vi "CPP-BLplotter.vi"(0 "Plot Array":cluster{dbl[], dbl[]}[](array[cluster])=[{[500.0, 500.0, 953.54, 215.0, 270.0, 320.0, 445.0, 525.0, 600.0, 675.0, 750.0, 825.0, 900.0, 960.0, 1010.0, 1060.0], [4.614524, 4.54365, 5.818368, 0.1374656, 0.6662545, 1.465458, 3.619824, 4.848976, 5.887329, 5.940571, 6.152151, 5.717487, 5.600293, 5.40069, 5.154843, 5.121789]}, {[100.0, 150.0, 215.0, 270.0, 320.0, 445.0, 525.0, 600.0, 675.0, 750.0, 825.0, 900.0, 960.0, 1010.0, 1060.0], [0.002314715, -0.00693192, 0.120417, 0.6880509, 1.519176, 3.513709, 5.065183, 6.116033, 6.096773, 5.938465, 5.593788, 5.5597, 5.387002, 5.304077, 4.887903]}] {"?" format="%.2f"; "?" format="%.2f"}, 1 "Job Directory":path=path "/G4_2_HD/Users/paulhayden/Documents/Projects/Westlakes_resolution") -> (2 "Saved Automatically?":bool, 3 "gnuplotScript":string="set term epslatex\nset output \"Plot.eps\"\nset xlabel '$Distance~(m)$'\nset ylabel '$DF~(s/m^3)\\times10^6$'\nset samples 1000\nset pointsize 1.00\nset title '$B38~Centreline~Glc$' 0, 0\nset size 0.75,0.9\n\n#set key 450, -2.5833\n unset key\nset label 1 '~~~~~~~~~~~Angle~(deg)~=~0' at -100, -2.58\nset label 2 '~~~~~~~~~~~Height~(m)~=~5' at -100, -3.27\n set xrange [0 : 500] \n# set autoscale x \n set yrange [0.10000 : 7]\n# set autoscale y \n\nplot \"B38_Centreline_Glc.dat\" index 0 using 1:2 axes x1y1 title '$File=B38R~DDD.xls$' with points 1 1, \\\n\"B38_Centreline_Glc.dat\" index 1 using 1:2 axes x1y1 title '$File=B38R~DDD~1.xls$' with points 1 3", 4 "Plot data file":path)   [LabVIEW 2012]
uses:
  Results_plotter_Global.vi
panel:
  in  "Tab Control":enum32{"Good Shit", "Boring Shit"}(tab)
  in  "Cancel Button":bool
  in  "Print Button":bool
  out "Velocity":cluster{dbl[], dbl[]}(graph)
  out "Turbulence":cluster{dbl[], dbl[]}(graph)
  in  "Plot Title":u16(ring) items=["Title String Only", "Number of Measurements", "Measuring:Instrument:Type", "Comments::", "Profile::", "URef::", "ULoc::", "HF:X:(mm)", "HF:Y:(mm)", "HF:Z:(mm)", "HF:DipAngle:Deg", "Uhf/Uref::", "TI:HF:%", "Uhf::", "Var(hf)::", "5HP:X:(mm)", "5HP:Y:(mm)", "5HP:Z:(mm)", "U5hp/Uref::", "V5hp/Uref::", "W5hp/Uref::", "Vmag5hp/Uref::", "TI:U5HP:%", "TI:V5HP:%", "TI:W5HP:%", "TI:Vmag5HP:%", "U_Mean::", "U_SD::", "V_Mean::", "V_SD::", "W_Mean::", "W_SD::", "Vmag_Mean::", "Vmag_SD::", "GoodFraction::", "5HP:P1:mmH2O", "Skew(hf)::", "Kurt(hf)::", "HF:Standard Error:in Mean", "HF:Standard Error:in Variance", "HF:Timescale Estimate:Integrated to 25%", "Reference:Temperature:Used for Corrections", "Atmos:Pressure:Used for Corrections", "Date::", "Multi Run:Start Time:", "Time:Measurement:Commenced", "Seconds:since:1st Jan", "Messages::", "Raw:Data:Filename"]
  in  "Filename Max length":i32=255
  out "Final Title":string="B38 Centreline Glc"
  out "Path":path
  in  "Plot Title Post Block":string
  in  "Plot Title Pre Block":string
  in  "Show Script Editor?":bool
  # "put a load of nice controls here for ref height etc, then a button to say \"print it\" that makes and runs a gnuplot script for \nthe graphs as you have them....."
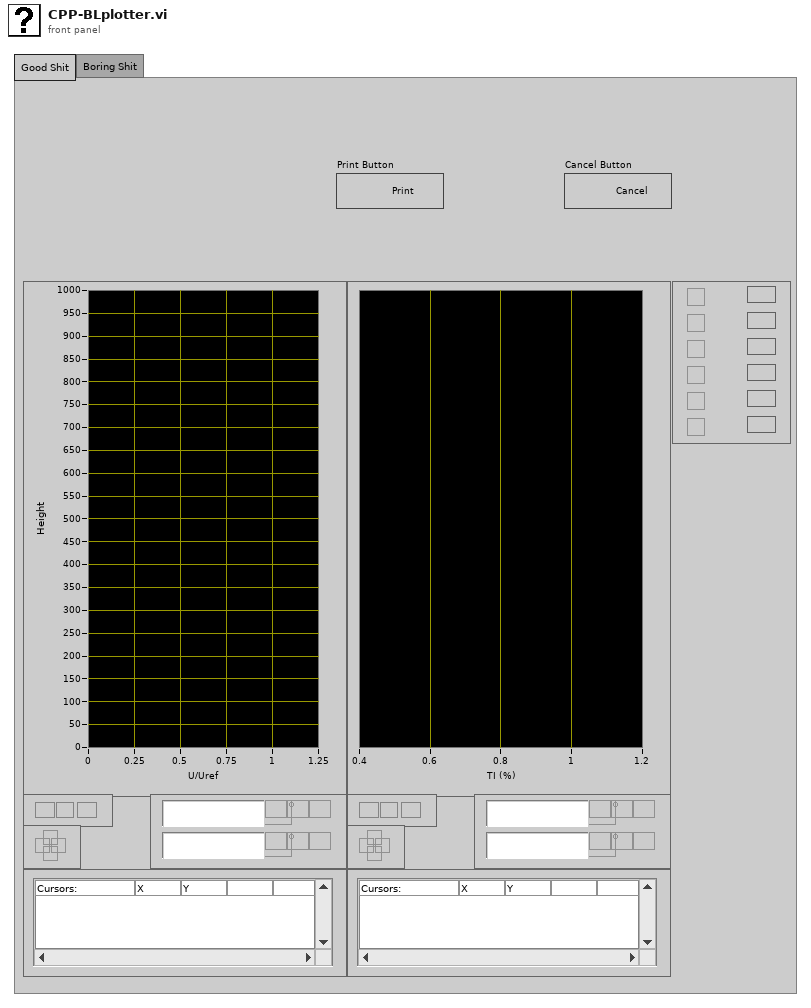
[diagram p1: front panel]
types:
  T1 = typedef "LVRangeTypeDef.ctl" = cluster{"Minimum":dbl, "Maximum":dbl, "Increment":dbl, "Minor Increment":dbl, "Start":dbl}
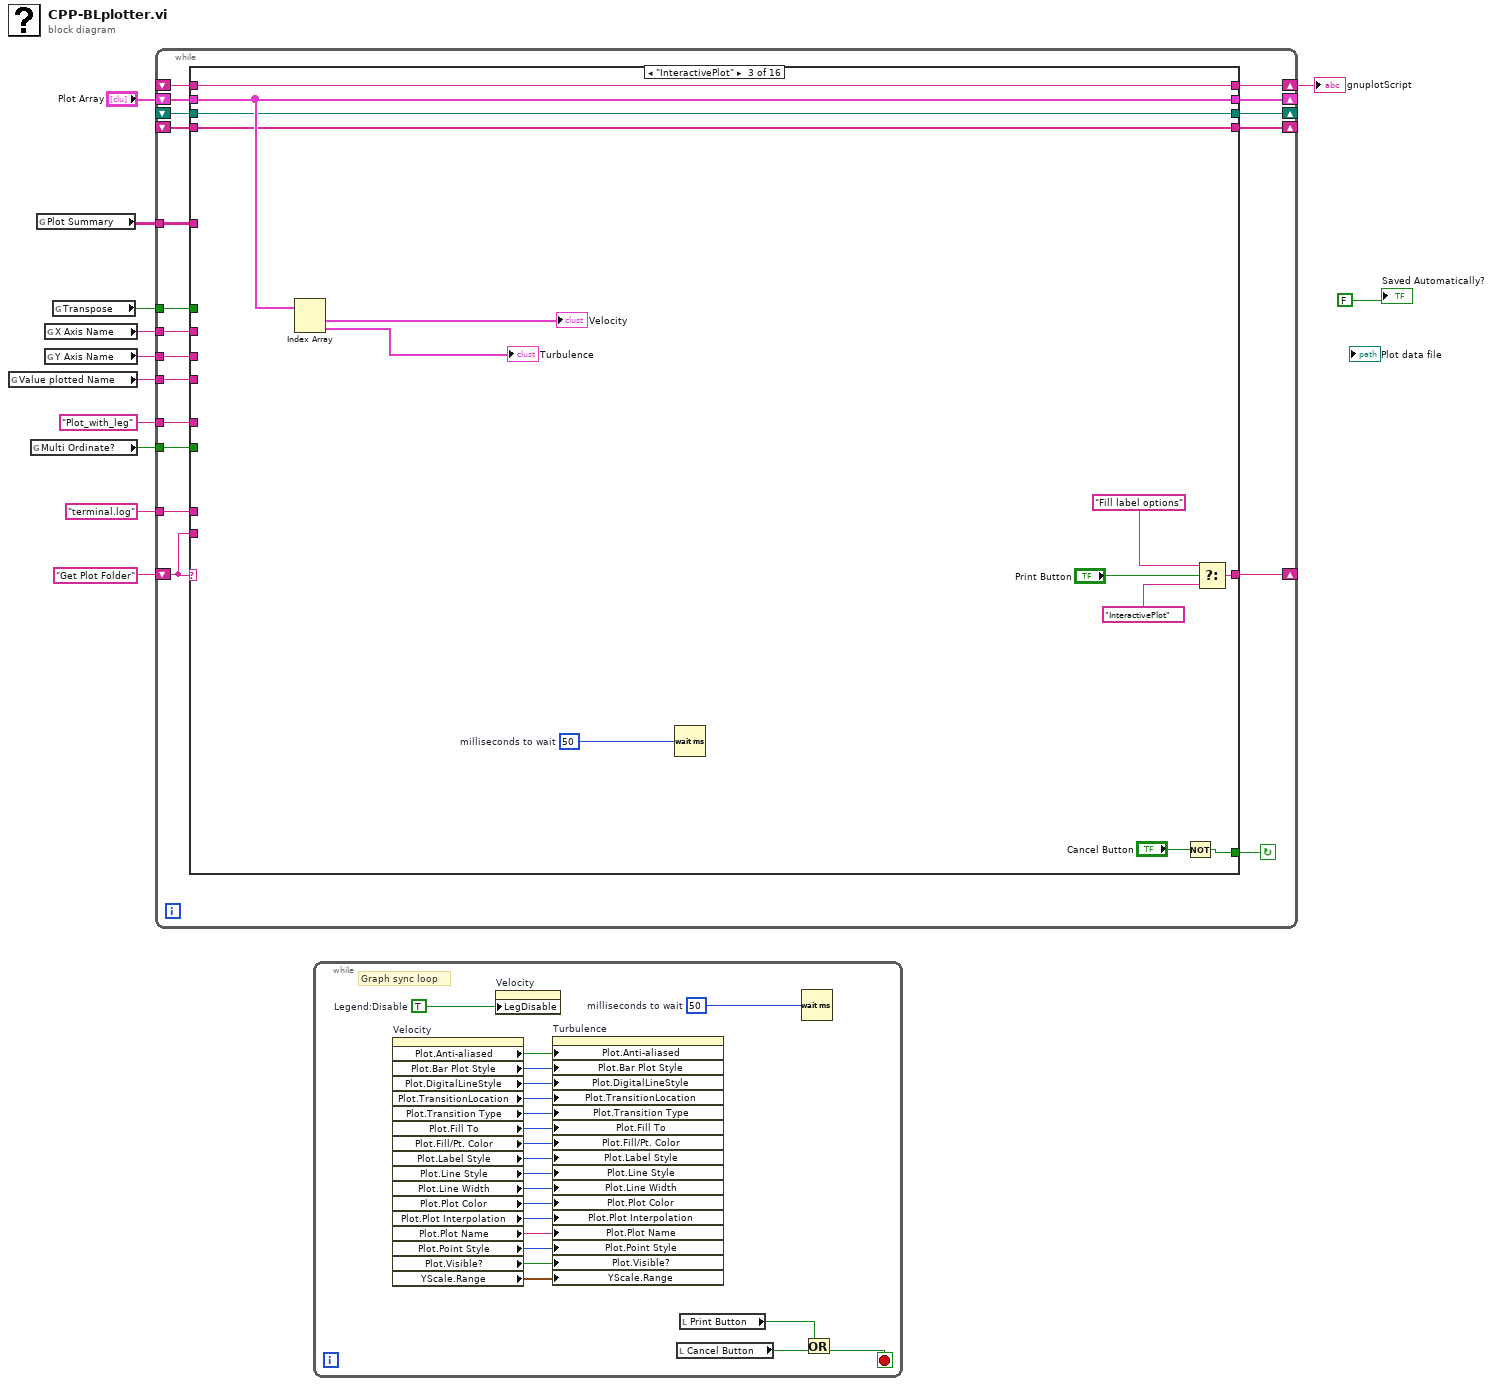
[diagram p0: block diagram]
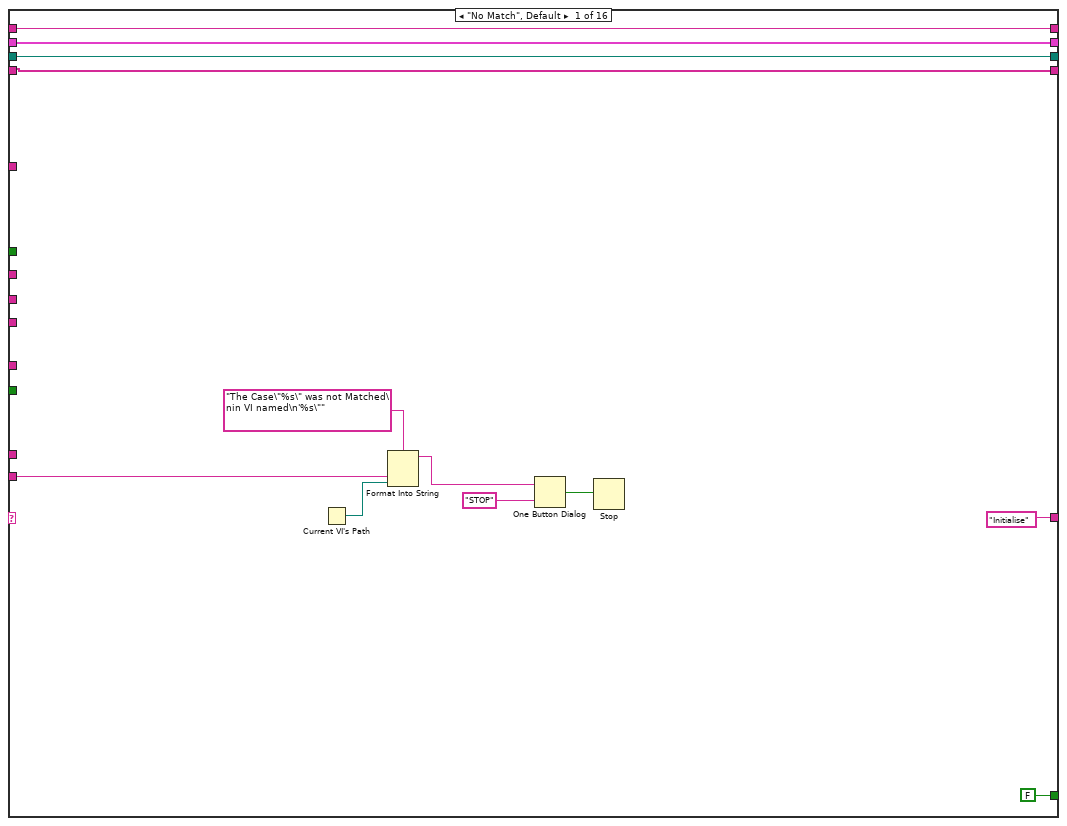
[diagram p2: hidden frame]
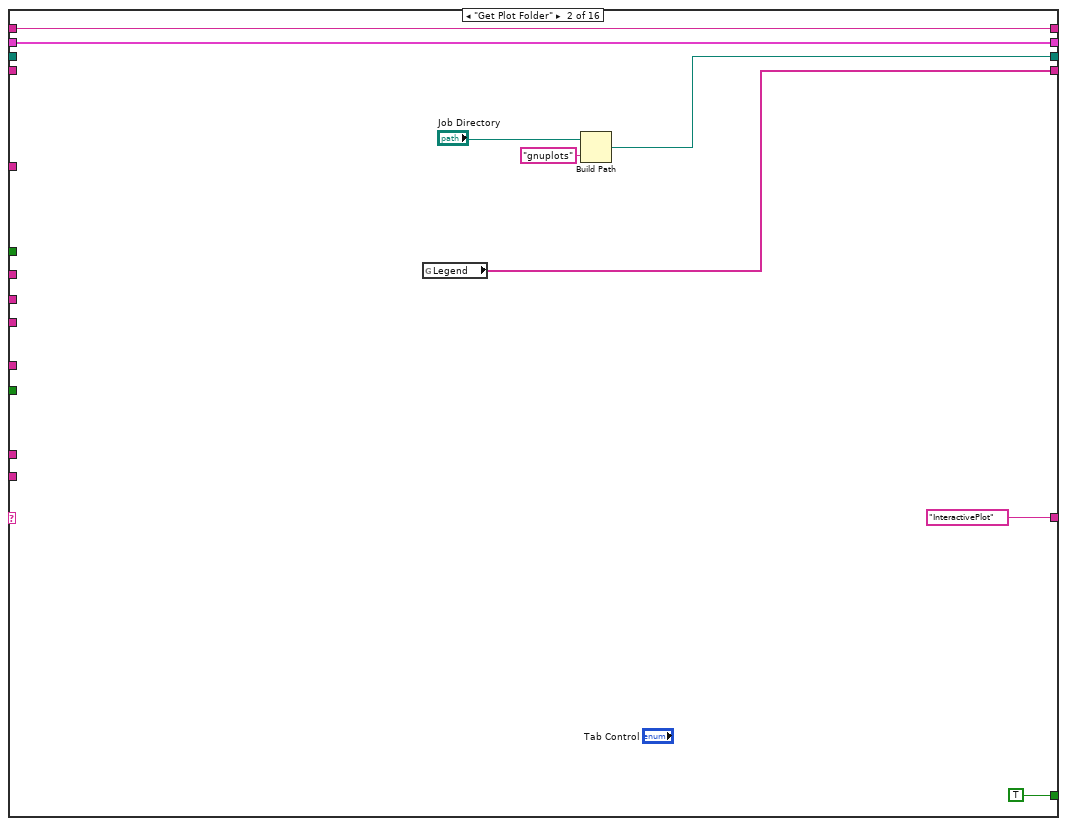
[diagram p3: hidden frame]
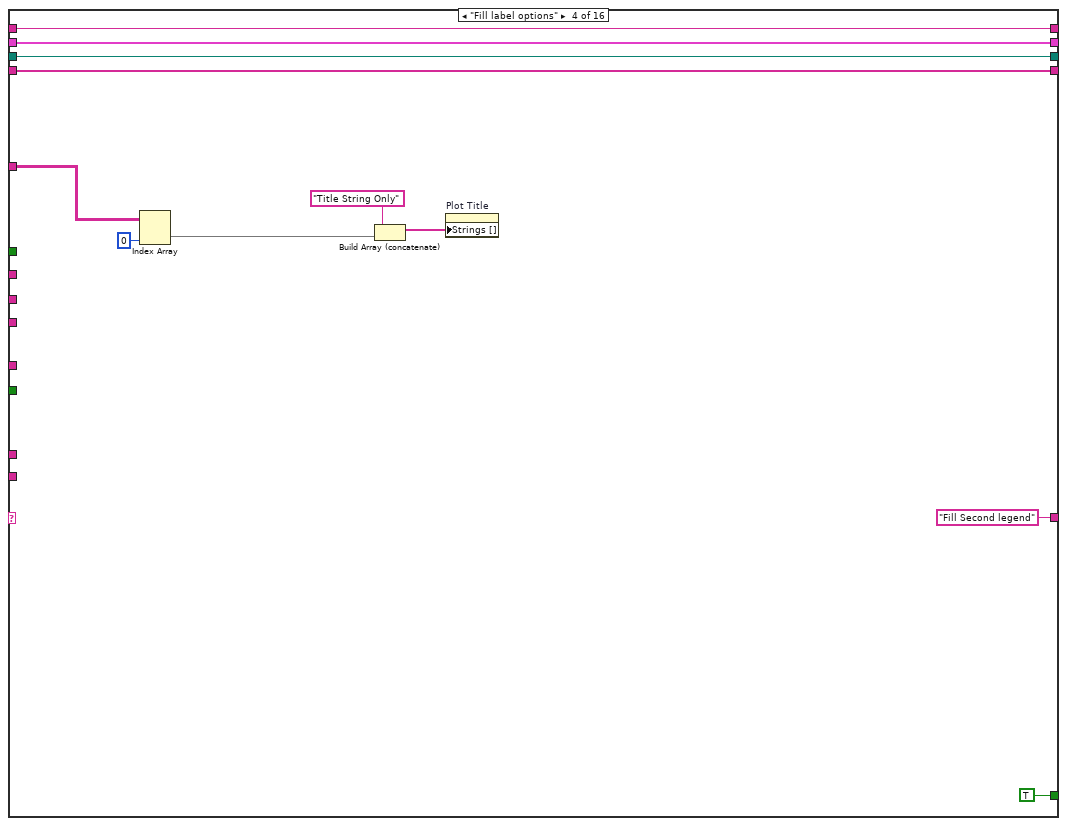
[diagram p4: hidden frame]
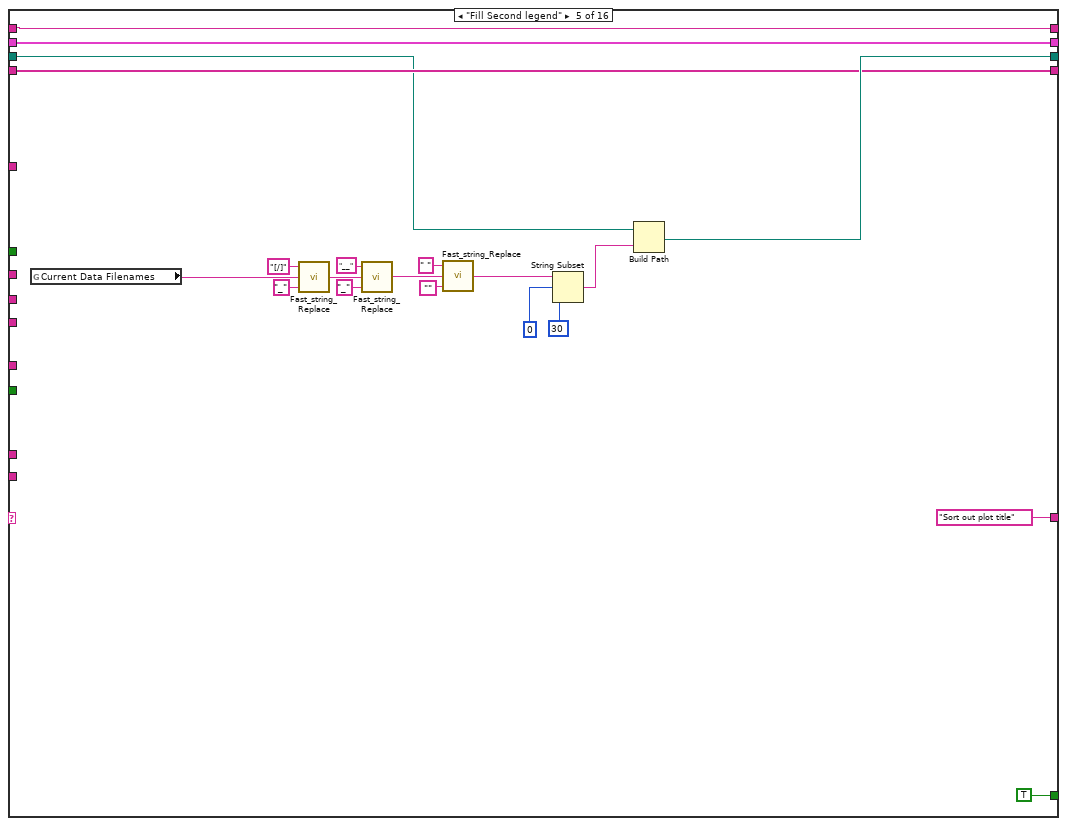
[diagram p5: hidden frame]
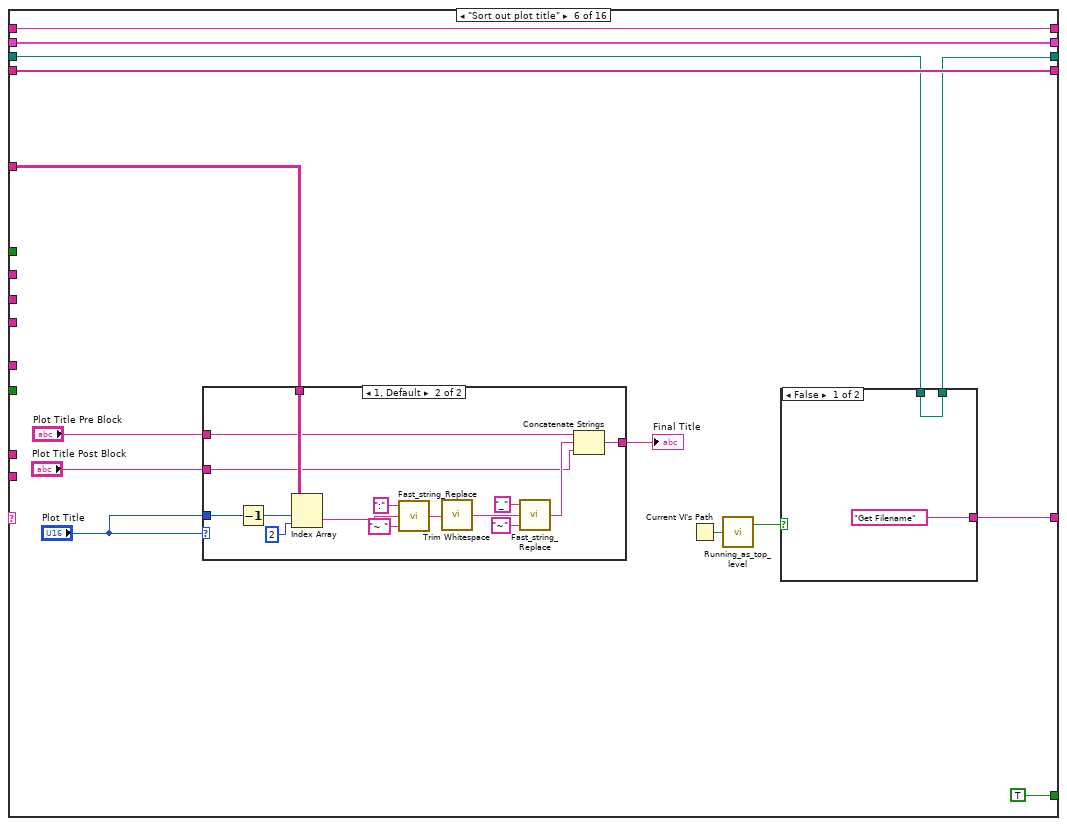
[diagram p6: hidden frame]
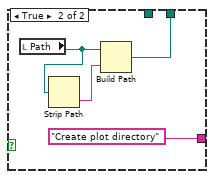
[diagram p7: hidden frame]
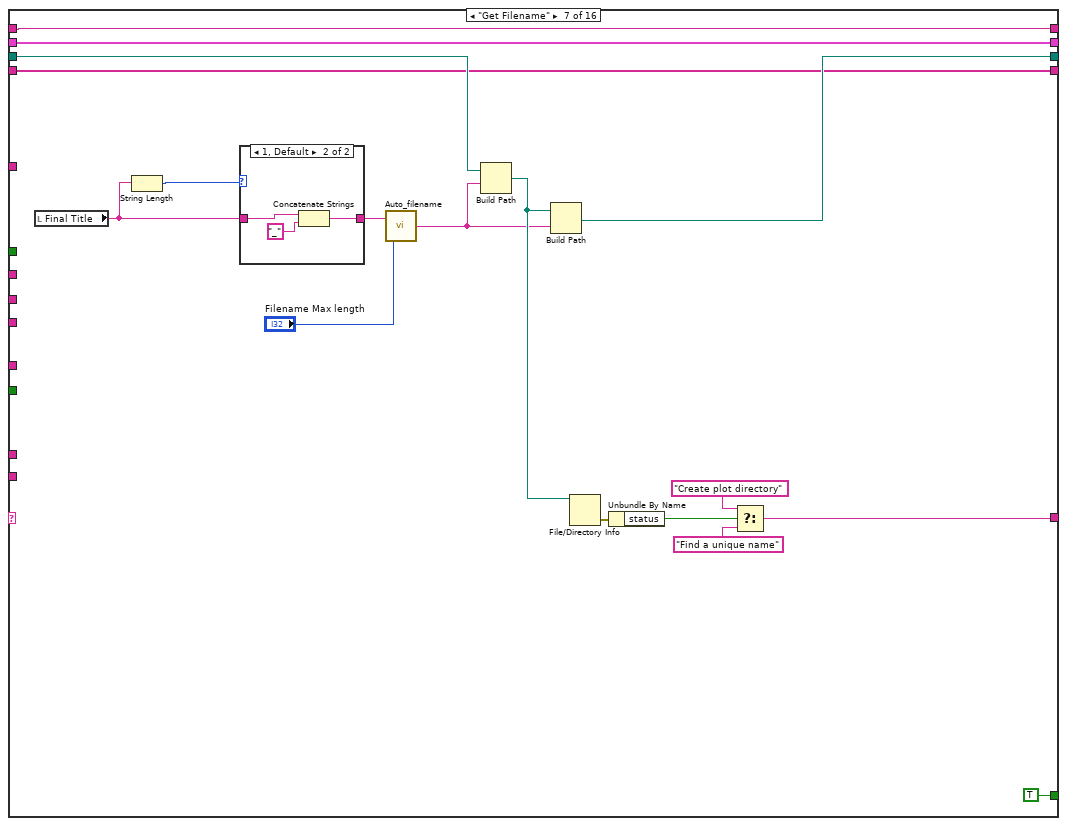
[diagram p9: hidden frame]
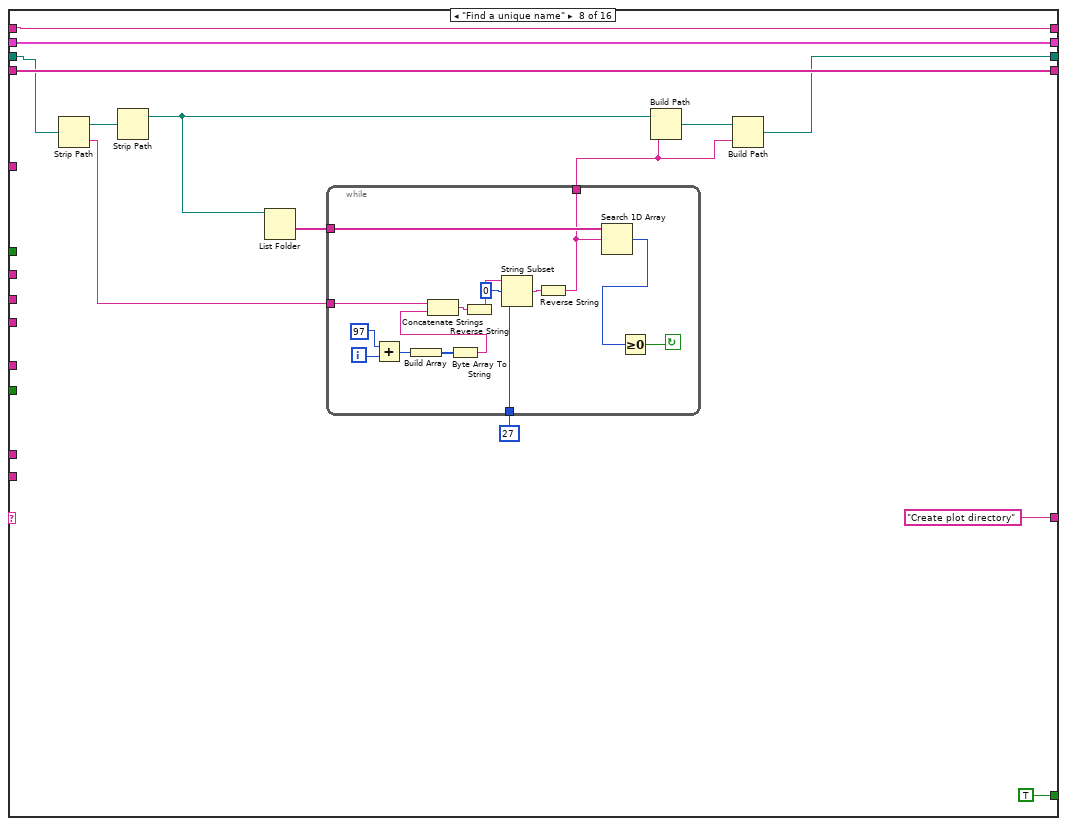
[diagram p11: hidden frame]
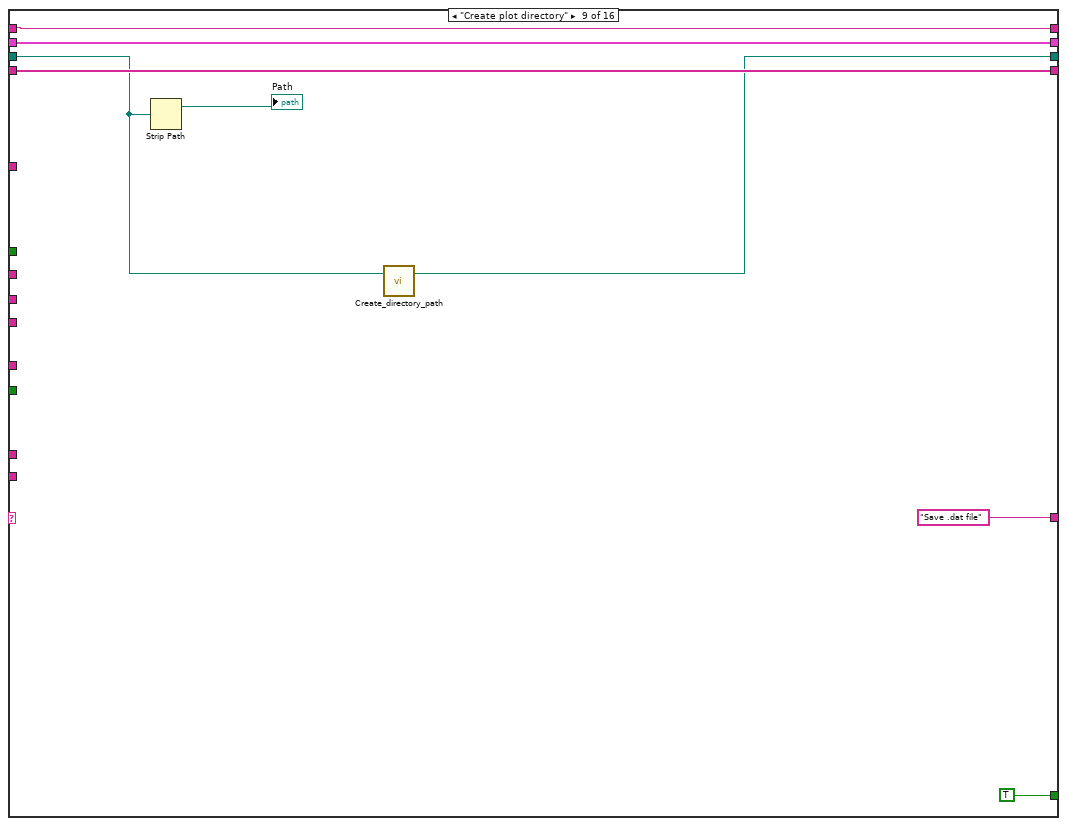
[diagram p12: hidden frame]
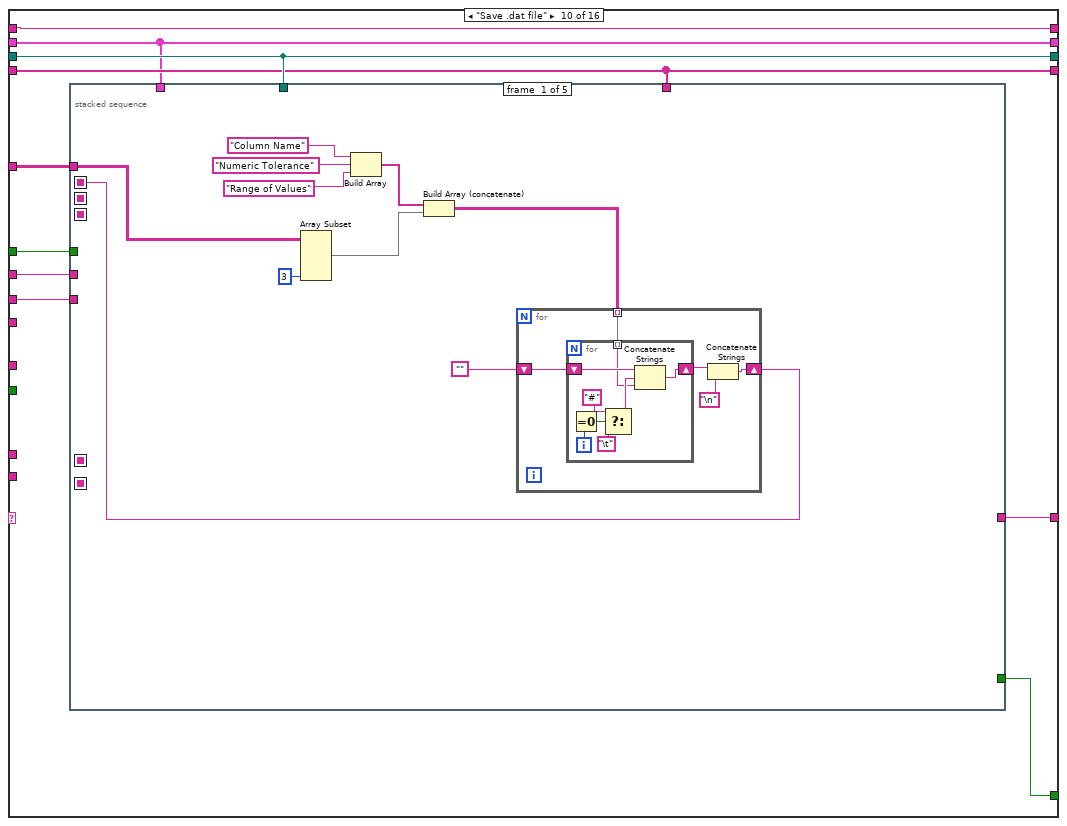
[diagram p13: hidden frame]
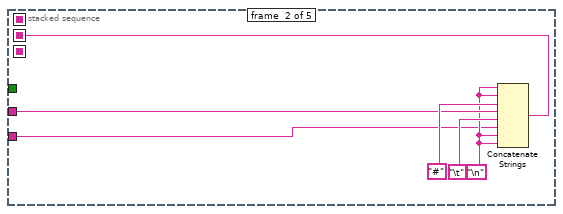
[diagram p14: hidden frame]
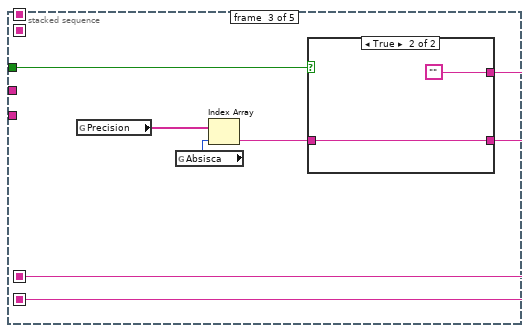
[diagram p15: hidden frame]
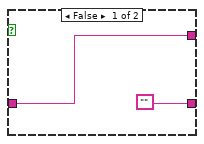
[diagram p16: hidden frame]
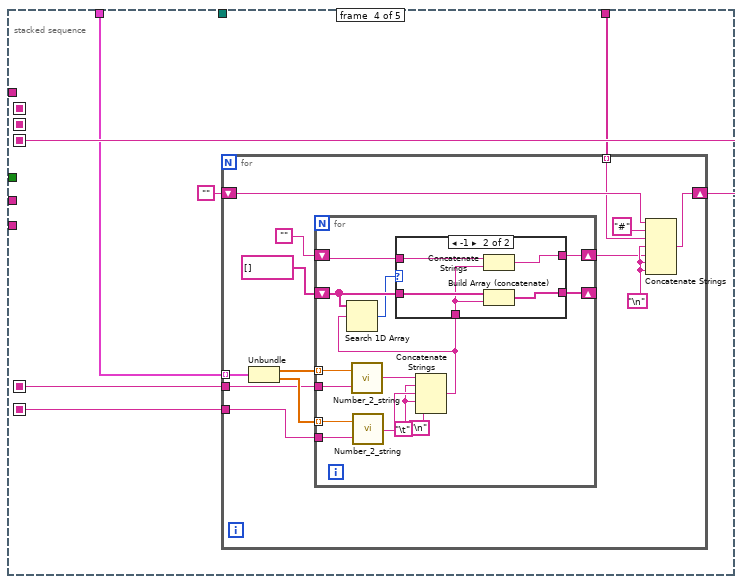
[diagram p17: hidden frame]
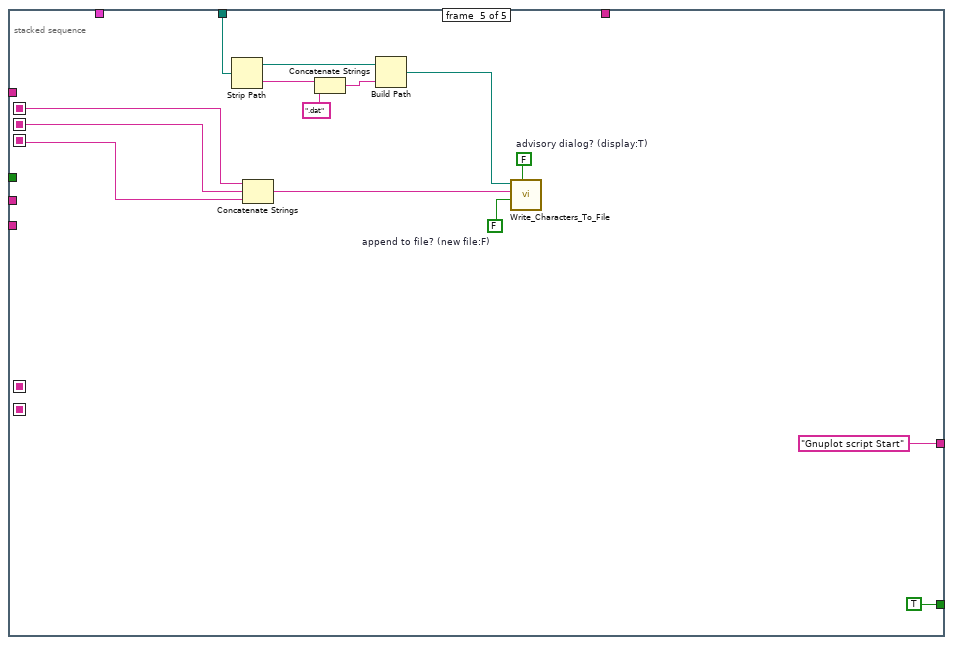
[diagram p19: hidden frame]
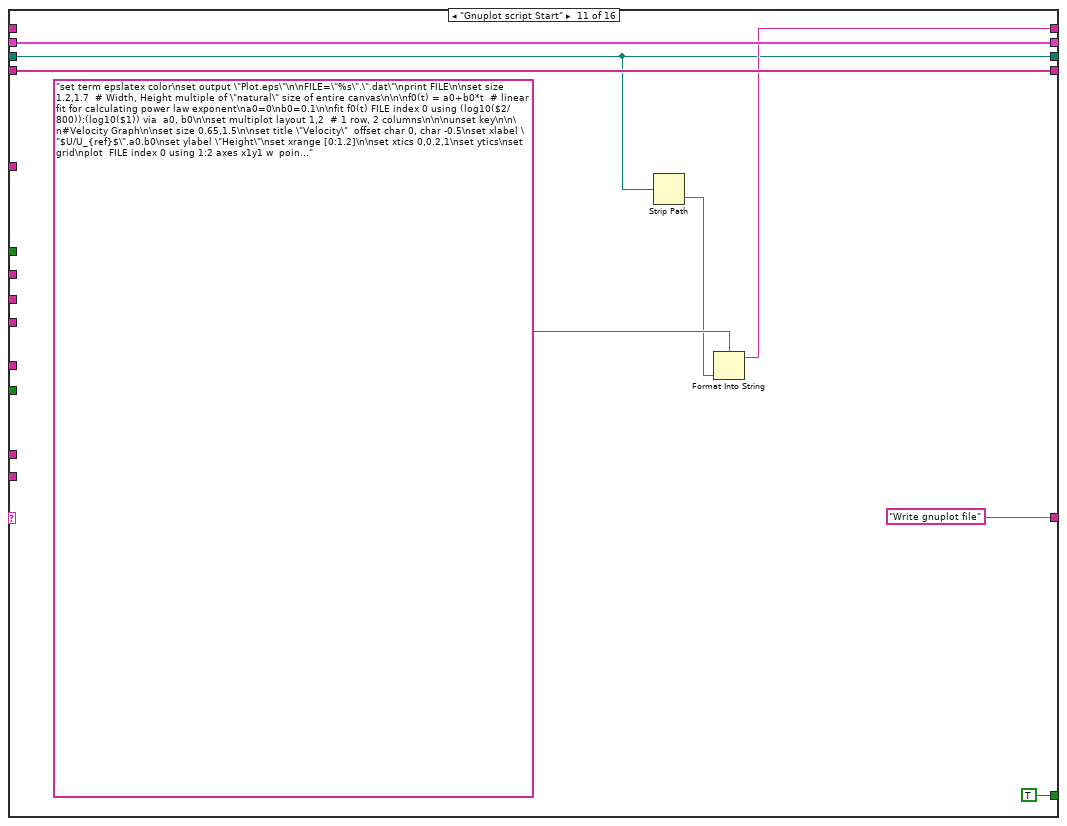
[diagram p20: hidden frame]
diagram:
  n1 = global read "Results_plotter_Global.vi" "Value plotted Name"() -> (w8:string)
  n2 = global read "Results_plotter_Global.vi" "Multi Ordinate?"() -> (w1:bool)
  n3 = global read "Results_plotter_Global.vi" "Plot Summary"() -> (w11:string[][])
  n4 = global read "Results_plotter_Global.vi" "X Axis Name"() -> (w10:string)
  n5 = global read "Results_plotter_Global.vi" "Y Axis Name"() -> (w9:string)
  n6 = global read "Results_plotter_Global.vi" "Transpose"() -> (w2:bool)
  n7 = while {
    shift-left: "Get Plot Folder" -> [w30]
    shift-right: [w13] -> _
    tunnel: w11 -> [w29]
    shift-right: [w28] -> _
    shift-left: _ -> [w27]
    tunnel: w10 -> [w26]
    tunnel: w9 -> [w25]
    tunnel: w8 -> [w24]
    shift-right: [w22] -> _
    shift-left: "Plot Array" -> [w23]
    shift-right: [w20] -> w7
    shift-left: _ -> [w21]
    tunnel: "Plot_with_leg" ("name or relative path") -> [w19]
    shift-right: [w18] -> _
    shift-left: _ -> [w17]
    tunnel: "terminal.log" -> [w16]
    tunnel: w2 -> [w15]
    tunnel: w1 -> [w14]
    stop <- w31 continue-if-true
    n8 = case shown="\"InteractivePlot\"" w30 {
      tunnel: [FALSE TRUE w53 TRUE ("Top Level") TRUE ("Top Level") TRUE ("Top Level") TRUE ("Top Level") TRUE ("Top Level") TRUE w197 TRUE ("Top Level") TRUE ("Top Level") TRUE ("Top Level") TRUE ("Top Level") FALSE ("Top Level") FALSE ("Top Level")] -> w31
      tunnel: ["Initialise" "InteractivePlot" w58 "Fill Second legend" "Sort out plot title" w97 w146 "Create plot directory" "Save .dat file" w196 "Write gnuplot file" ("t") "Execute shell script" ("t") "Has pdf been generated?" ("t") w320 "End" "End" ("t")] -> w13
      tunnel: w30 -> [w38 _ _ _ _ _ _ _ _ _ _ _ _ _ _ _]
      tunnel: w29 -> [_ _ _ w75 _ w104 _ _ _ w195 _ _ _ _ _ _]
      tunnel: [w35 w48 w61 w69 w95 w99 w147 w153 w186 w198 w295 w305 w313 w324 w329 w339] -> w28
      tunnel: w27 -> [w35 _ w61 w69 w91 w98 w143 w160 w185 w198 w295 w305 w313 w324 w329 w339]
      tunnel: w26 -> [_ _ _ _ _ _ _ _ _ w194 _ _ _ _ _ _]
      tunnel: w25 -> [_ _ _ _ _ _ _ _ _ w193 _ _ _ _ _ _]
      tunnel: w24 -> [_ _ _ _ _ _ _ _ _ _ _ _ _ _ _ _]
      tunnel: w23 -> [w34 w45 w62 w70 w94 w109 w145 w163 w189 w190 w300 w311 w318 w327 w334 w344]
      tunnel: [w34 w45 w62 w70 w94 w109 w145 w163 w189 w190 w300 w311 w318 w327 w334 w344] -> w22
      tunnel: w21 -> [w33 w47 w59 w71 w93 w105 w144 w162 w188 w199 _ w301 w316 w325 w332 w342]
      tunnel: [w33 w47 w59 w71 w93 w105 w144 w162 w188 w199 w296 w301 w316 w325 w332 w342] -> w20
      tunnel: w19 -> [_ _ _ _ _ _ _ _ _ _ _ _ _ _ _ _]
      tunnel: [w32 w44 w60 w68 w92 w108 w142 w161 w187 w192 w299 w306 w317 w326 w333 w343] -> w18
      tunnel: w17 -> [w32 _ w60 w68 w92 w108 w142 w161 w187 w192 w299 w306 w317 w326 w333 w343]
      tunnel: w16 -> [_ _ _ _ _ _ _ _ _ _ _ _ w312 _ _ w337]
      tunnel: w15 -> [_ _ _ _ _ _ _ _ _ w191 _ _ _ _ _ _]
      tunnel: w14 -> [_ _ _ _ _ _ _ _ _ _ _ _ _ _ _ _]
      frame "No Match", Default {
        n9 = Current VI's Path() -> (path=w37:path)
        n10 = Format Into String(format string="The Case\"%s\" was not Matched\nin VI named\n'%s\"" ("Format String"), w38, w37) -> (resulting string=w41:string)  [unwired: 2 in, 1 out]
        n11 = One Button Dialog(message=w41, button name ("OK")="STOP") -> (true=w39:bool)
        n12 = Stop(stop? (T)=w39) -> ()
      }
      frame "Get Plot Folder" {
        n13 = global read "Results_plotter_Global.vi" "Legend"() -> (w44:string[])
        n14 = Build Path(base path="Job Directory", name or relative path="gnuplots") -> (appended path=w48:path)
      }
      frame "InteractivePlot" {
        w52 = u32 50  # milliseconds to wait
        n15 = Index Array(array=w62) -> (element #1=→"Velocity":cluster{dbl[], dbl[]}, element #2=→"Turbulence":cluster{dbl[], dbl[]})  [unwired: 2 in]
        n16 = Wait (ms)(milliseconds to wait=w52) -> ()  [unwired: 1 out]
        n17 = Not(x="Cancel Button") -> (.not. x?=w53:bool)
        n18 = Select(t="Fill label options", s="Print Button", f="InteractivePlot") -> (s? t:f=w58:string)
      }
      frame "Fill label options" {
        n19 = Index Array(array=w75, index (col)=0 ("disabled index (col)")) -> (element=w66:string[])  [unwired: 1 in]
        n20 = Build Array (concatenate)("Title String Only", w66) -> (w65:string[])
        n21 = property on="Plot Title" class="Ring (strict)"("Strings []"=w65) -> ()  [unwired: 2 in, 2 out]
      }
      frame "Fill Second legend" {
        n22 = global read "Results_plotter_Global.vi" "Current Data Filenames"() -> (w80:string)
        n23 = call "Fast_string_Replace.vi"("Replace match with:"="_", "Input String"=w80, "regular expression"="[/]") -> ("Output String"=w84:string)  [unwired: 2 out]
        n24 = call "Fast_string_Replace.vi"("Replace match with:"="_", "Input String"=w84, "regular expression"="__") -> ("Output String"=w81:string)  [unwired: 2 out]
        n25 = call "Fast_string_Replace.vi"("Replace match with:"="", "Input String"=w81, "regular expression"=" ") -> ("Output String"=w79:string)  [unwired: 2 out]
        n26 = String Subset(string=w79, offset (0)=0, length (rest)=30 ("length (rest)")) -> (substring=w78:string)
        n27 = Build Path(base path=w91, name or relative path=w78) -> (appended path=w95:path)
      }
      frame "Sort out plot title" {
        n28 = case shown="1, Default" "Plot Title" {
          tunnel: [w116 w121] -> w103
          tunnel: "Plot Title Pre Block" -> [w116 w120]
          tunnel: w104 -> [_ w124]
          tunnel: "Plot Title" -> [_ w123]
          tunnel: "Plot Title Post Block" -> [_ w117]
          frame 0 {
          }
          frame 1, Default {
            n29 = Decrement(x=w123) -> (x-1=w122:u16)
            n30 = Index Array(array=w124, index (row)=w122, index (col)=u16 2 ("y")) -> (element=w127:string)
            n31 = call "Fast_string_Replace.vi"("Replace match with:"="~ ", "Input String"=w127, "regular expression"=":") -> ("Output String"=w126:string)  [unwired: 2 out]
            n32 = call <vilib>:"Trim Whitespace.vi"("string"=w126) -> ("trimmed string"=w125:string)  [unwired: 1 in]
            n33 = call "Fast_string_Replace.vi"("Replace match with:"="~", "Input String"=w125, "regular expression"="_") -> ("Output String"=w119:string)  [unwired: 2 out]
            n34 = Concatenate Strings(w120, w119, w117) -> (w121:string)
          }
        }
        "Final Title" <- w103
        n35 = Current VI's Path() -> (path=w102:path)
        n36 = call "Running_as_top_level.vi"("Vi path name"=w102) -> ("Top Level"=w100:bool)  [unwired: 1 out]
        n37 = case shown="False" w100 {
          tunnel: [w111 w114] -> w99
          tunnel: w98 -> [w111 _]
          tunnel: ["Get Filename" ("t") "Create plot directory"] -> w97
          frame False {
          }
          frame True {
            n38 = local read "Path"() -> (w113:path)
            n39 = Strip Path(path=w113) -> (name=w112:string)  [unwired: 1 out]
            n40 = Build Path(base path=w113, name or relative path=w112) -> (appended path=w114:path)
          }
        }
      }
      frame "Get Filename" {
        n41 = local read "Final Title"() -> (w132:string)
        n42 = String Length(string=w132) -> (length=w134:i32)
        n43 = case shown="1, Default" w134 {
          tunnel: [w149 w150] -> w133
          tunnel: w132 -> [w149 w152]
          frame 0 {
          }
          frame 1, Default {
            n44 = Concatenate Strings(w152, "_") -> (w150:string)
          }
        }
        n45 = call "Auto_filename.vi"("Filename Max length"="Filename Max length", "Prefix"=w133) -> ("Filename"=w136:string)
        n46 = Build Path(base path=w143, name or relative path=w136) -> (appended path=w140:path)
        n47 = Build Path(base path=w140, name or relative path=w136) -> (appended path=w147:path)
        n48 = File/Directory Info(path=w140) -> (error out=w141:errorcluster)  [unwired: 1 in, 6 out]
        n49 = Unbundle By Name(w141) -> ("status"=w139:bool)
        n50 = Select(t="Create plot directory", s=w139, f="Find a unique name") -> (s? t:f=w146:string)
      }
      frame "Find a unique name" {
        n51 = Strip Path(path=w160) -> (stripped path=w159:path, name=w158:string)
        n52 = Strip Path(path=w159) -> (stripped path=w156:path)  [unwired: 1 out]
        n53 = List Folder(path=w156) -> (folder names=w157:string[])  [unwired: 1 in, 5 out]
        n54 = while {
          tunnel: w158 -> [w181]
          tunnel: 27 ("Max Length") -> [w180]
          tunnel: [w169] -> w155
          tunnel: w157 -> [w170]
          i -> [w171]
          stop <- w167 continue-if-true
          n55 = Add(x=97, y=w171) -> (x+y=w178:i32)
          n56 = Build Array(w178) -> (w179:i32[])
          n57 = Byte Array To String(unsigned byte array=w179) -> (string=w176:string)
          n58 = Concatenate Strings(w181, w176) -> (w174:string)
          n59 = Reverse String(1:w174) -> (0:w175:string)
          n60 = String Subset(string=w175, offset (0)=0, length (rest)=w180) -> (substring=w173:string)
          n61 = Reverse String(1:w173) -> (0:w169:string)
          n62 = Search 1D Array(1D array=w170, element=w169) -> (index of element=w168:i32)  [unwired: 1 out]
          n63 = Greater Or Equal To 0?(x=w168) -> (x >= 0?=w167:bool)
        }
        n64 = Build Path(base path=w156, name or relative path=w155) -> (appended path=w154:path)
        n65 = Build Path(base path=w154, name or relative path=w155) -> (appended path=w153:path)
      }
      frame "Create plot directory" {
        n66 = Strip Path(path=w185) -> (stripped path=→"Path":path)  [unwired: 1 out]
        n67 = call "Create_directory_path.vi"("Path name"=w185) -> ("Path name Out"=w186:path)  [unwired: 1 in, 1 out]
      }
      frame "Save .dat file" {
        n68 = stacked-sequence {
          seq-local: [w200 _ _ _ _] -> [_ _ _ _ w284]
          seq-local: [_ w224 _ _ _] -> [_ _ _ _ w285]
          seq-local: [_ _ _ w243 _] -> [_ _ _ _ w286]
          seq-local: [_ _ w229 _ _] -> [_ _ _ w241 _]
          seq-local: [_ _ w231 _ _] -> [_ _ _ w240 _]
          tunnel: w198 -> [_ _ _ _ w289]
          tunnel: [_ _ _ _ TRUE ("Top Level")] -> w197
          tunnel: [_ _ _ _ "Gnuplot script Start"] -> w196
          tunnel: w195 -> [w205 _ _ _ _]
          tunnel: w194 -> [_ w227 _ _ _]
          tunnel: w193 -> [_ w223 _ _ _]
          tunnel: w190 -> [_ _ _ w239 _]
          tunnel: w192 -> [_ _ _ w242 _]
          tunnel: w191 -> [_ _ w232 _ _]
          frame #0 {
            n69 = Array Subset(array=w205, length (col)=3 ("length")) -> (w203:string[][])  [unwired: 3 in]
            n70 = Build Array("Column Name", "Numeric Tolerance", "Range of Values") -> (w209:string[])
            n71 = Build Array (concatenate)(w209, w203) -> (w201:string[][])
            n72 = for {
              shift-right: [w213] -> w200
              shift-left: "" -> [w210]
              tunnel: w201 -> [w214] mode=indexing
              n73 = for {
                shift-right: [w215] -> w212
                shift-left: w210 -> [w222]
                tunnel: w214 -> [w216] mode=indexing
                i -> [w221]
                n74 = Equal To 0?(x=w221) -> (x = 0?=w220:bool)
                n75 = Select(t="#", s=w220, f="\t") -> (s? t:f=w217:string)
                n76 = Concatenate Strings(w222, w217, w216) -> (w215:string)
              }
              n77 = Concatenate Strings(w212, "\n") -> (w213:string)
            }
          }
          frame #1 {
            w225 = "\n"
            n78 = Concatenate Strings(w225, w225, "#" ("string"), w227, "\t", w223, w225, w225) -> (w224:string)
          }
          frame #2 {
            n79 = global read "Results_plotter_Global.vi" "Precision"() -> (w234:string[])
            n80 = global read "Results_plotter_Global.vi" "Absisca"() -> (w233:i32)
            n81 = Index Array(array=w234, index=w233) -> (element=w230:string)
            n82 = case shown="True" w232 {
              tunnel: ["" w238] -> w231
              tunnel: w230 -> [w235 w238]
              tunnel: [w235 ""] -> w229
              frame False {
              }
              frame True {
              }
            }
          }
          frame #3 {
            n83 = for {
              tunnel: w239 -> [w257] mode=indexing
              shift-right: [w256] -> w243
              shift-left: "" -> [w250]
              tunnel: w242 -> [w248] mode=indexing
              tunnel: w241 -> [w246]
              tunnel: w240 -> [w245]
              w255 = "\n"
              n84 = Unbundle(w257) -> (w251:dbl[], w252:dbl[])
              n85 = for {
                tunnel: w251 -> [w271] mode=indexing
                shift-right: [w266] -> w254
                shift-left: "" -> [w267]
                tunnel: w252 -> [w259] mode=indexing
                shift-right: [w265] -> _
                shift-left: string[] [] -> [w264]
                tunnel: w246 -> [w261]
                tunnel: w245 -> [w260]
                w268 = "\t"
                n86 = call "Number_2_string.vi"("precision"=w261, "number"=w271) -> ("String"=w270:string)
                n87 = call "Number_2_string.vi"("precision"=w260, "number"=w259) -> ("String"=w269:string)
                n88 = Concatenate Strings(w270, w268, w269, w268, "\n") -> (w263:string)
                n89 = Search 1D Array(1D array=w264, element=w263) -> (index of element=w262:i32)  [unwired: 1 in]
                n90 = case shown="-1" w262 {
                  tunnel: w267 -> [w273 w278]
                  tunnel: [w273 w277] -> w266
                  tunnel: w263 -> [_ w274]
                  tunnel: w264 -> [w272 w276]
                  tunnel: [w272 w275] -> w265
                  frame 0, Default {
                  }
                  frame -1 {
                    n91 = Concatenate Strings(w278, w274) -> (w277:string)
                    n92 = Build Array (concatenate)(w276, w274) -> (w275:string[])
                  }
                }
              }
              n93 = Concatenate Strings(w250, "#", w248, w255, w254, w255, w255) -> (w256:string)
            }
          }
          frame #4 {
            w281 = FALSE  # advisory dialog? (display:T)
            w282 = FALSE  # append to file? (new file:F)
            n94 = Strip Path(path=w289) -> (stripped path=w290:path, name=w292:string)
            n95 = Concatenate Strings(w284, w285, w286) -> (w283:string)
            n96 = Concatenate Strings(w292, ".dat" ("string")) -> (w291:string)
            n97 = Build Path(base path=w290, name or relative path=w291) -> (appended path=w280:path)
            n98 = call "Write_Characters_To_File.vi"("file path (dialog if empty)"=w280, "advisory dialog? (display:T)"=w281, "character string"=w283, "append to file? (new file:F)"=w282) -> ()  [unwired: 1 in, 4 out]
          }
        }
      }
      frame "Gnuplot script Start" {
        n99 = Strip Path(path=w295) -> (name=w293:string)  [unwired: 1 out]
        n100 = Format Into String(format string="set term epslatex color\nset output \"Plot.eps\"\n\nFILE=\"%s\".\".dat\"\nprint FILE\n\nset size 1.2,1.7  # Width, Height multiple of \"natural\" size of entire canvas\n\n\nf0(t) = a0+b0*t  # linear fit for calculating power law exponent\na0=0\nb0=0.1\n\nfit f0(t) FILE index 0 using (log10($2/800)):(log10($1)) via  a0, b0\n\nset multiplot layout 1,2  # 1 row, 2 columns\n\n\nunset key\n\n\n#Velocity Graph\n\nset size 0.65,1.5\n\nset title \"Velocity\"  offset char 0, char -0.5\nset xlabel \"$U/U_{ref}$\".a0.b0\nset ylabel \"Height\"\nset xrange [0:1.2]\n\nset xtics 0,0.2,1\nset ytics\nset grid\nplot  FILE index 0 using 1:2 axes x1y1 w  points lc 0 pointtype 4 pointsize 1, f0(x) w lines\n\n#Turbulence Graph\n\nset size 0.55,1.5\nset origin 0.65,0\n\nset title \"Turbulence\"  offset char 0, char -0.5\nset xlabel \"$TI$\"\nunset ylabel\nset xrange [0:35]\n\nset format y \"\"\nset xtics 5,5\nset ytics\nset grid\nplot  FILE index 1 using 1:2 axes x1y1 w  points lc 1 pointtype 4 pointsize 1\n\n\n\nunset multiplot\n", w293) -> (resulting string=w296:string)  [unwired: 2 in, 1 out]
      }
      frame "Write gnuplot file" {
        w308 = FALSE  # append to file? (new file:F)
        w309 = FALSE  # advisory dialog? (display:T)
        n101 = Strip Path(path=w305) -> (stripped path=w302:path)  [unwired: 1 out]
        n102 = Build Path(base path=w302, name or relative path="gnuplot_script.txt") -> (appended path=w310:path)
        n103 = call "Write_Characters_To_File.vi"("file path (dialog if empty)"=w310, "advisory dialog? (display:T)"=w309, "character string"=w301, "append to file? (new file:F)"=w308) -> ()  [unwired: 1 in, 4 out]
      }
      frame "Execute shell script" {
        n104 = call "Run_Gnuplot_Script.vi"("logfileName"=w312, "workingDirectory"=w313) -> ()
      }
      frame "Has pdf been generated?" {
        n105 = Select(t="Show Re-Run Gnuplot?", s="Show Script Editor?", f="Open Standard output file") -> (s? t:f=w320:string)
      }
      frame "Show Re-Run Gnuplot?" {
        n106 = Strip Path(path=w329) -> (stripped path=w328:path)  [unwired: 1 out]
        n107 = call "Re_run_Gnuplot.vi"("Plot folder (dialog if empty)"=w328) -> ()  [unwired: 4 out]
      }
      frame "Open Standard output file" {
        n108 = Strip Path(path=w339) -> (stripped path=w336:path)  [unwired: 1 out]
        n109 = Format Into String(format string="open \"%s\"", w337) -> (resulting string=w335:string)  [unwired: 2 in, 1 out]
        n110 = call <vilib>:"System Exec.vi"("working directory"=w336, "command line"=w335) -> ()  [unwired: 4 in, 6 out]
      }
    }
  }
  "gnuplotScript" <- w7
  n111 = while {
    stop <- w348 stop-if-true
    w345 = TRUE  # Legend:Disable
    w346 = u32 50  # milliseconds to wait
    # "Graph sync loop"
    n112 = property on="Velocity" class="XYGraph (strict)"() -> ("Plot.Anti-aliased"=w365:bool, "Plot.Bar Plot Style"=w364:u8, "Plot.DigitalLineStyle"=w363:u8, "Plot.TransitionLocation"=w362:u8, "Plot.Transition Type"=w361:u8, "Plot.Fill To"=w360:i16, "Plot.Fill/Pt. Color"=w359:u32, "Plot.Label Style"=w358:u8, "Plot.Line Style"=w357:u8, "Plot.Line Width"=w356:u8, "Plot.Plot Color"=w355:u32, "Plot.Plot Interpolation"=w354:u8, "Plot.Plot Name"=w353:string, "Plot.Point Style"=w352:u8, "Plot.Visible?"=w351:bool, "YScale.Range"=w350:T1)  [unwired: 2 in, 2 out]
    n113 = property on="Velocity" class="XYGraph (strict)"("LegDisable"=w345) -> ()  [unwired: 2 in, 2 out]
    n114 = property on="Turbulence" class="XYGraph (strict)"("Plot.Anti-aliased"=w365, "Plot.Bar Plot Style"=w364, "Plot.DigitalLineStyle"=w363, "Plot.TransitionLocation"=w362, "Plot.Transition Type"=w361, "Plot.Fill To"=w360, "Plot.Fill/Pt. Color"=w359, "Plot.Label Style"=w358, "Plot.Line Style"=w357, "Plot.Line Width"=w356, "Plot.Plot Color"=w355, "Plot.Plot Interpolation"=w354, "Plot.Plot Name"=w353, "Plot.Point Style"=w352, "Plot.Visible?"=w351, "YScale.Range"=w350) -> ()  [unwired: 2 in, 2 out]
    n115 = local read "Cancel Button"() -> (w349:bool)
    n116 = local read "Print Button"() -> (w347:bool)
    n117 = Wait (ms)(milliseconds to wait=w346) -> ()  [unwired: 1 out]
    n118 = Or(x=w347, y=w349) -> (x .or. y?=w348:bool)
  }
  "Saved Automatically?" <- FALSE
